vi "libssh2_knownhost_get - no previous - returns first host.vi"() -> ()   [LabVIEW 2013, in "libssh2_tests.lvlib"]
uses:
  libssh2_tests.lvlib
  libssh2/libssh2_init_default.vi
  <vilib>/addons/_JKI Toolkits/Caraya/classes/Assert/Assert Equal Value_Variant.vi
  <vilib>/addons/_JKI Toolkits/Caraya/classes/Test/Test.lvclass
  libssh2/libssh2.lvlib
  <vilib>/addons/_JKI Toolkits/Caraya/classes/Assert/Assert.lvclass
panel:
  out "error out":errorcluster
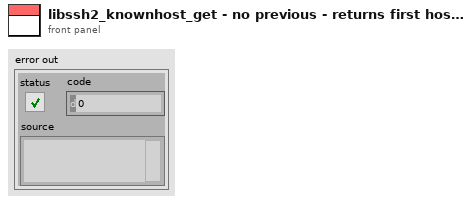
[diagram p1: front panel]
types:
  T1 = typedef "libssh2.lvlib/Session Refnum.ctl" = refnum<k1>
  T2 = typedef "libssh2.lvlib/Known Host Collection Refnum.ctl" = refnum<k1>
  T3 = typedef "libssh2.lvlib/Known Host Refnum.ctl" = refnum<k1>
  T4 = typedef "libssh2.lvlib/libssh2_knownhost.ctl" = cluster{"magic":u32, "node":u64, "name":string, "key":string, "typemask":i32}
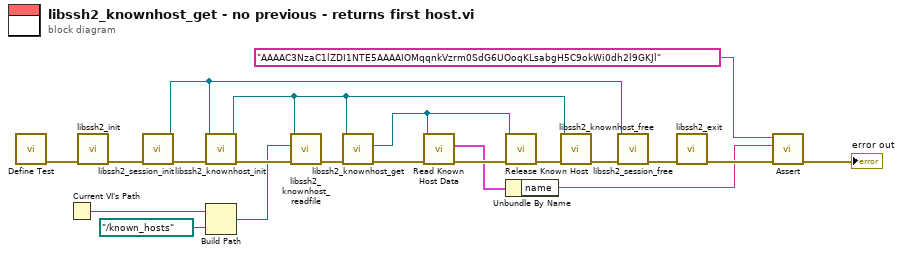
[diagram p0: block diagram]
diagram:
  n1 = call <vilib>:"Define Test.vi"() -> ("error out"=w20:errorcluster)  [unwired: 10 in, 1 out]
  n2 = Current VI's Path() -> (path=w11:path)
  n3 = call-poly "libssh2_init.vi"("error in (no error)"=w20) -> ("error out"=w19:errorcluster)  [unwired: 10 in]
  n4 = call "libssh2_session_init.vi"("error in (no error)"=w19) -> ("error out"=w18:errorcluster, "session"=w15:T1)  [unwired: 9 in]
  n5 = call "libssh2_knownhost_init.vi"("error in (no error)"=w18, "session"=w15) -> ("error out"=w13:errorcluster, "known hosts collection"=w8:T2)  [unwired: 8 in]
  n6 = Build Path(base path=w11, name or relative path=path "../known_hosts" ("filename")) -> (appended path=w9:path)
  n7 = call "libssh2_knownhost_readfile.vi"("error in (no error)"=w13, "filename"=w9, "known hosts collection"=w8) -> ("error out"=w12:errorcluster)  [unwired: 7 in, 1 out]
  n8 = call "libssh2_knownhost_get.vi"("error in (no error)"=w12, "known hosts collection"=w8) -> ("error out"=w6:errorcluster, "next"=w4:T3)  [unwired: 7 in, 1 out]
  n9 = call "Read Known Host Data.vi"("error in (no error)"=w6, "known host"=w4) -> ("error out"=w5:errorcluster, "known host data"=w3:T4)  [unwired: 8 in]
  n10 = call "Release Known Host.vi"("error in (no error)"=w5, "known host"=w4) -> ("error out"=w7:errorcluster)  [unwired: 9 in]
  n11 = Unbundle By Name(w3) -> ("name"=w2:string)
  n12 = call "libssh2_knownhost_free.vi"("error in (no error)"=w7, "known hosts collection"=w8) -> ("error out"=w14:errorcluster)  [unwired: 9 in]
  n13 = call "libssh2_session_free.vi"("error in (no error)"=w14, "session"=w15) -> ("error out"=w17:errorcluster)  [unwired: 9 in]
  n14 = call "libssh2_exit.vi"("error in (no error)"=w17) -> ("error out"=w16:errorcluster)  [unwired: 10 in]
  n15 = call-poly <vilib>:"Assert.vi"("error in (no error)"=w16, "Y"=w2, "X"="AAAAC3NzaC1lZDI1NTE5AAAAIOMqqnkVzrm0SdG6UOoqKLsabgH5C9okWi0dh2l9GKJl" ("key")) -> ("error out"=→"error out":errorcluster)  [unwired: 7 in, 1 out]
